vi "FindMassResolution_Array.vi"(10 "Signal":cluster{"m/z Array":dbl[], "Signal":sgl[]}) -> (1 "FWHM":dbl, 2 "Resolution":dbl)   [LabVIEW 2013]
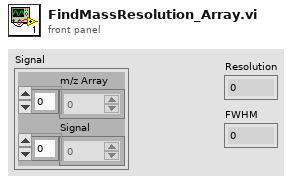
[diagram p1: front panel]
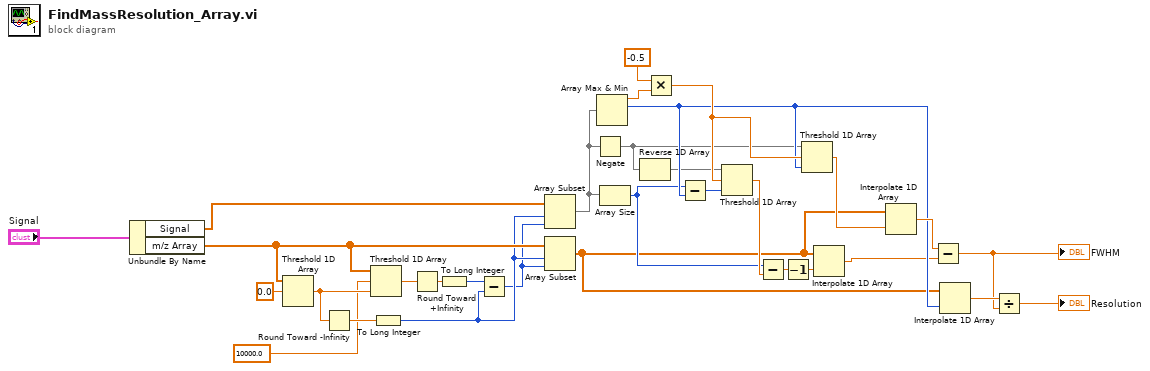
[diagram p0: block diagram]
diagram:
  n1 = Unbundle By Name("Signal") -> ("Signal"=w23:sgl[], "m/z Array"=w20:dbl[])
  n2 = Threshold 1D Array(2:0.0 ("threshold y"), 3:w20) -> (0:w27:dbl)  [unwired: 1 in]
  n3 = Round Toward -Infinity(1:w27) -> (0:w29:dbl)
  n4 = Threshold 1D Array(1:w27, 2:10000.0 ("threshold y"), 3:w20) -> (0:w31:dbl)
  n5 = To Long Integer(number=w29) -> (32bit integer=w19:i32)
  n6 = Round Toward +Infinity(x=w31) -> (ceil(x): smallest int >= x=w30:dbl)
  n7 = To Long Integer(number=w30) -> (32bit integer=w28:i32)
  n8 = Subtract(x=w28, y=w19) -> (x-y=w18:i32)
  n9 = Array Subset(array=w23, index=w19, length=w18) -> (w13:sgl[])
  n10 = Array Subset(array=w20, index=w19, length=w18) -> (w7:dbl[])
  n11 = Negate(x=w13) -> (-x=w5:sgl[])
  n12 = Array Max & Min(array=w13) -> (max value=w26:sgl, max index (indices)=w11:i32)  [unwired: 2 out]
  n13 = Array Size(array=w13) -> (size(s)=w8:i32)
  n14 = Reverse 1D Array(array=w5) -> (reversed array=w6:sgl[])
  n15 = Multiply(x=-0.5, y=w26) -> (x*y=w15:dbl)
  n16 = Subtract(x=w8, y=w11) -> (x-y=w12:i32)
  n17 = Threshold 1D Array(1:w12, 2:w15, 3:w6) -> (0:w16:sgl)
  n18 = Subtract(x=w8, y=w16) -> (x-y=w9:sgl)
  n19 = Decrement(x=w9) -> (x-1=w4:sgl)
  n20 = Threshold 1D Array(1:w11, 2:w15, 3:w5) -> (0:w17:sgl)
  n21 = Interpolate 1D Array(1:w4, 2:w7) -> (0:w10:dbl)
  n22 = Interpolate 1D Array(1:w17, 2:w7) -> (0:w24:dbl)
  n23 = Subtract(x=w24, y=w10) -> (x-y=w21:dbl)
  "FWHM" <- w21
  n24 = Interpolate 1D Array(1:w11, 2:w7) -> (0:w22:dbl)
  n25 = Divide(x=w22, y=w21) -> (x/y=→"Resolution":dbl)
